vi "Add Monitor Channel.vi"(8 "error in":errorcluster, 10 "Channel Array":string[](array[string]), 11 "Section Ptr in":T1 format="%.0x") -> (0 "error out":errorcluster, 2 "Channel Refs":T1[](array[typedef]) format="%.0x", 3 "Section Ptr out":T1 format="%.0x")   [LabVIEW 2020, in "AIM ARINC 664 Scripting.lvlib"]
uses:
  AIM ARINC 664 Scripting.lvlib
  <vilib>/NI VeriStand/Custom Device API/Custom Device Item Ref.ctl
  <vilib>/NI VeriStand/Custom Device API/Custom Device Channel.ctl
  <vilib>/NI VeriStand/Custom Device API/Custom Device Channel Type.ctl
  <vilib>/NI VeriStand/Custom Device API/Custom Device API.lvlib
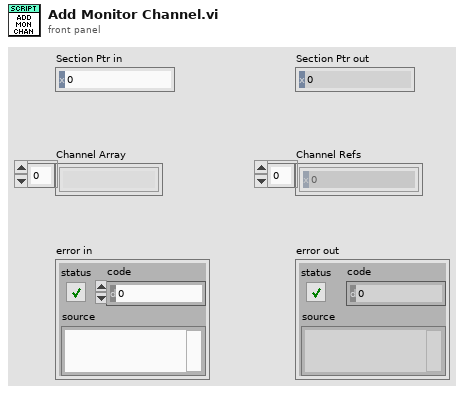
[diagram p1: front panel]
types:
  T1 = typedef "Custom Device API.lvlib/Custom Device Item Ref.ctl" = u64
  T2 = typedef "Custom Device API.lvlib/Custom Device Channel.ctl" = cluster{"Type":T3, "Units":string, "Default Value":dbl, "Faultable":bool, "Scalable":bool}
  T3 = typedef "Custom Device API.lvlib/Custom Device Channel Type.ctl" = enum16{"Input", "Output"}
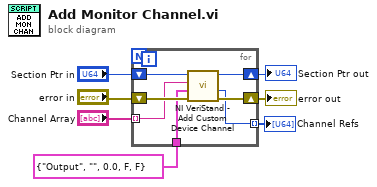
[diagram p0: block diagram]
diagram:
  n1 = for {
    tunnel: [w10] -> w1 mode=indexing
    shift-right: [w11] -> w7
    shift-left: "error in" -> [w14]
    tunnel: "Channel Array" -> [w8] mode=indexing
    tunnel: T2 {"Type"=enum."Output", "Units"="", "Default Value"=0.0, "Faultable"=FALSE, "Scalable"=FALSE} ("Channel") -> [w9]
    shift-right: [w13] -> w6
    shift-left: "Section Ptr in" -> [w12]
    n2 = call <vilib>:"NI VeriStand - Add Custom Device Channel.vi"("error in (no error)"=w14, "Channel"=w9, "Channel Name"=w8, "Parent Ref in"=w12) -> ("error out"=w11:errorcluster, "Channel Ref"=w10:T1, "Parent Ref out"=w13:T1)  [unwired: 4 in, 1 out]
  }
  "error out" <- w7
  "Section Ptr out" <- w6
  "Channel Refs" <- w1
